vi "Stopping.vi"(6 "Teller":T1 {"AbsoluteTime" format="%<%x %.3X>T"}, 8 "Error in":errorcluster, 11 "Base Actor in":refnum<class "Base Actor.lvclass">) -> (0 "Error out":errorcluster, 3 "Base Actor out":refnum<class "Base Actor.lvclass">)   [LabVIEW 2020, in "jettl.lvlib" / "BaseActor.lvlib" / "Base Actor.lvclass"]
doc: "jettl 6.12.1.94\nNathan Davis - Nathan Davis\nCopyright (c) 2026, Nathan Davis\nMIT"
uses:
  Base Actor.lvclass
  Base Actor.lvclass/Base Actor.ctl
  jettl.lvlib
  ActorRelation.ctl
  MessageMetadata.ctl
  ActorLifetime.ctl
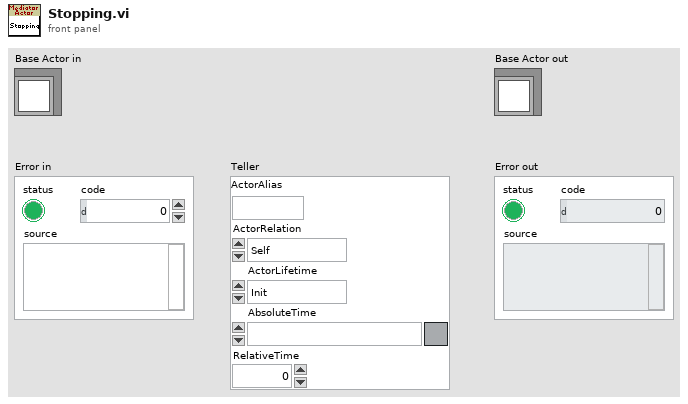
[diagram p1: front panel]
types:
  T1 = typedef "jettl.lvlib/MessageMetadata.ctl" = cluster{"ActorAlias":string, "ActorRelation":T2, "ActorLifetime":T3, "AbsoluteTime":timestamp, "RelativeTime":dbl}
  T2 = typedef "jettl.lvlib/ActorRelation.ctl" = enum16{"Self", "Mediator", "Component"}
  T3 = typedef "jettl.lvlib/ActorLifetime.ctl" = enum16{"Init", "Spawn", "Setup", "Teardown Before Running", "Running", "Stop Called", "Stopping With Children", "Stopping Without Children", "Teardown After Running", "Stopped"}
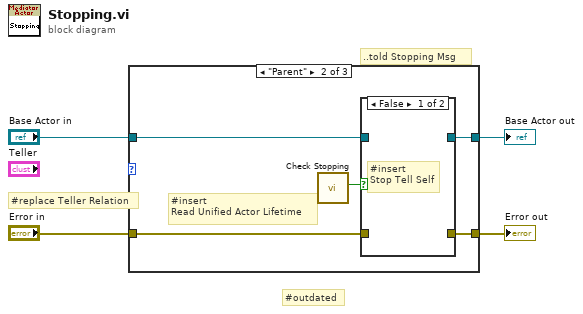
[diagram p0: block diagram]
diagram:
  # "#outdated"
  # "#replace Teller Relation"
  # "..told Stopping Msg"
  n1 = case shown="\"Parent\"" {
    selector: _ -> [_ _ _]
    tunnel: "Base Actor in" -> [w6 w8 w19]
    tunnel: [w6 w12 w19] -> w3
    tunnel: "Error in" -> [w5 w11 w18]
    tunnel: [w5 w10 w18] -> w1
    frame "Self" {
      # "Case will not fundamentally execute"
    }
    frame "Parent" {
      # "#insert\nRead Unified Actor Lifetime"
      n2 = call "Check Stopping.vi"() -> ("Stopping"=w9:bool, "Unified Actor Lifetime"=w7:T3)  [unwired: 10 in]
      n3 = case shown="False" w9 {
        tunnel: [w15 w17] -> w12
        tunnel: w11 -> [w14 w16]
        tunnel: [_ w16] -> w10
        tunnel: w8 -> [w13 w17]
        frame False {
          # "#insert\nStop Tell Self"
        }
        frame True {
        }
      }
    }
    frame "Child" {
      # "Case will not fundamentally execute"
    }
  }
  "Base Actor out" <- w3
  "Error out" <- w1
